vi "New.vi"(8 "Error In":errorcluster) -> (0 "Error Out":errorcluster, 3 "Parser":refnum<class "Parser.lvclass">)   [LabVIEW 2018, in "Toolkit.lvlib" / "Parser.lvclass"]
uses:
  Parser.lvclass
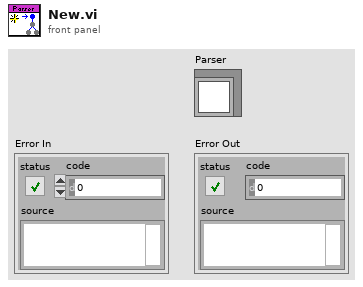
[diagram p1: front panel]
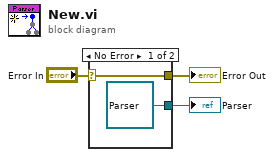
[diagram p0: block diagram]
diagram:
  n1 = case shown="No Error" "Error In" {
    selector: "Error In" -> [w4 w6]
    tunnel: [refnum<class "Parser.lvclass"> refnum ("Toolkit.lvlib:Parser.lvclass") _] -> w3
    tunnel: [w4 w6] -> w1
    frame No Error {
    }
    frame Error {
    }
  }
  "Parser" <- w3
  "Error Out" <- w1
